vi "testError.vi"() -> ()   [LabVIEW 2016]
uses:
  Controls/errorType.ctl
  ElectrometerError.lvclass
panel:
  in  "errorCode":i32
  out "Error":T1
  out "error out":errorcluster
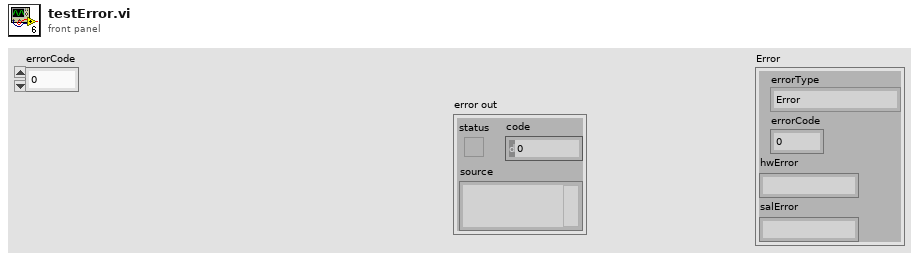
[diagram p1: front panel]
types:
  T1 = typedef "ElectrometerError.lvclass/errorType.ctl" = cluster{"errorType":enum16{"Error", "Warning", "None"}, "errorCode":dbl, "hwError":string, "salError":string}
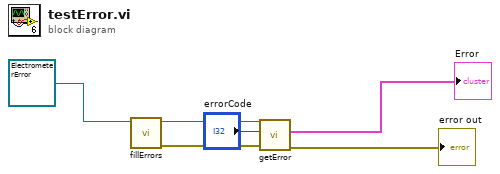
[diagram p0: block diagram]
diagram:
  n1 = call-dynamic "fillErrors.vi"("ElectrometerError in"=refnum<class "ElectrometerError.lvclass"> refnum) -> ("error out"=w4:errorcluster, "ElectrometerError out"=w5:refnum<class "ElectrometerError.lvclass">)  [unwired: 9 in]
  n2 = call-dynamic "getError.vi"("error in (no error)"=w4, "errorCode"="errorCode", "ElectrometerError in"=w5) -> ("error out"=→"error out":errorcluster, "Error"=→"Error":T1)  [unwired: 6 in, 1 out]
